vi "Processes_check.vi"(1 "검색 내용":string) -> (0 "불리언":bool)   [LabVIEW 2014]
panel:
  out "원소의 인덱스":i32
  in  "OpenVIs":bool
  out "Array":string[](array[string])
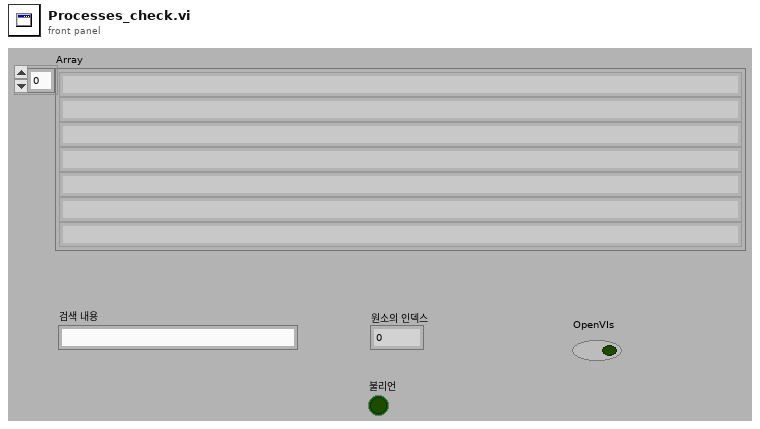
[diagram p1: front panel]
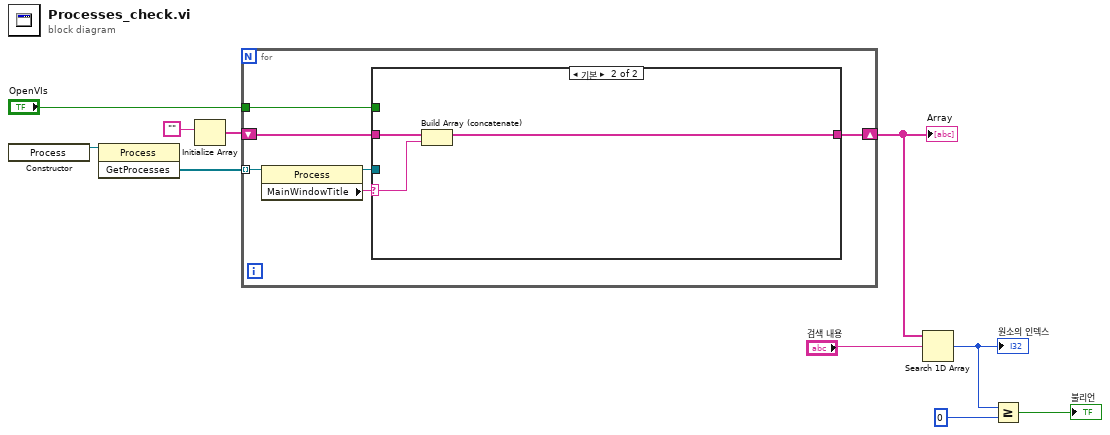
[diagram p0: block diagram]
diagram:
  n1 = constructor class="Process"() -> (reference out=w10:refnum<k24>)  [unwired: 3 in, 2 out]
  n2 = invoke class="Process" method="GetProcesses"(reference=w10) -> ("GetProcesses"=w9:refnum<k24>[])  [unwired: 2 in, 2 out]
  n3 = Initialize Array("") -> (w8:string[])  [unwired: 1 in]
  n4 = for {
    tunnel: w9 -> [w12] mode=indexing
    shift-right: [w15] -> w5
    shift-left: w8 -> [w16]
    tunnel: "OpenVIs" -> [w11]
    n5 = property class="Process"(reference=w12) -> (reference out=w14:refnum<k24>, "MainWindowTitle"=w13:string)  [unwired: 1 in, 1 out]
    n6 = case shown="기본" w13 {
      selector: w13 -> [_ w18]
      tunnel: w16 -> [w17 w20]
      tunnel: [w17 w19] -> w15
      tunnel: w14 -> [_ _]
      tunnel: w11 -> [_ _]
      frame "" {
      }
      frame Default {
        n7 = Build Array (concatenate)(w20, w18) -> (w19:string[])
      }
    }
  }
  "Array" <- w5
  n8 = Search 1D Array(1D array=w5, element="검색 내용") -> (index of element=w3:i32)  [unwired: 1 in]
  "원소의 인덱스" <- w3
  n9 = Greater Or Equal?(x=w3, y=0) -> (x >= y?=→"불리언":bool)
